vi "Wave2D_Cal U_Apply Corner.vi"(6 "time step":i32, 8 "y length":i32, 9 "x length":i32, 10 "Corner":T1, 11 "U In":dbl[][](array[numeric])) -> (3 "U Out":dbl[][](array[numeric]))   [LabVIEW 2020, in "NI_PDE.lvlib"]
uses:
  <vilib>/gmath/NI_PDE.lvlib
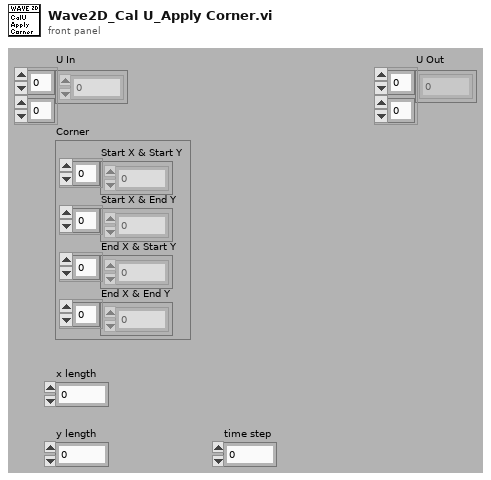
[diagram p1: front panel]
types:
  T1 = cluster{"Start X & Start Y":dbl[], "Start X & End Y":dbl[], "End X & Start Y":dbl[], "End X & End Y":dbl[]}
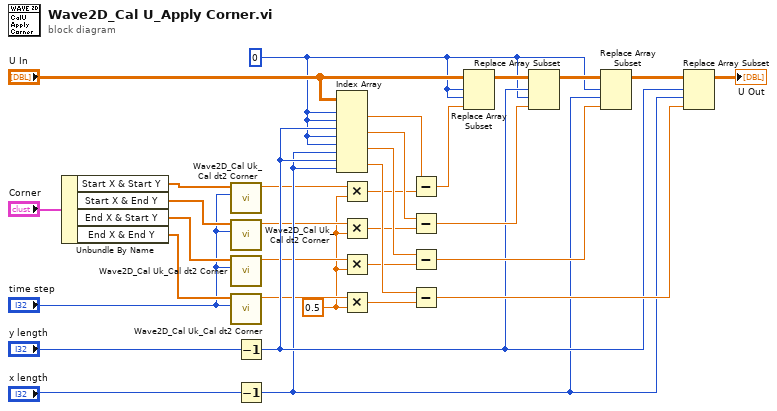
[diagram p0: block diagram]
diagram:
  w1 = 0.5 ("y")
  w11 = 0 ("index (row)")
  n1 = Unbundle By Name("Corner") -> ("Start X & Start Y"=w32:dbl[], "Start X & End Y"=w31:dbl[], "End X & Start Y"=w30:dbl[], "End X & End Y"=w29:dbl[])
  n2 = call <vilib>:"Wave2D_Cal Uk_Cal dt2 Corner.vi"("time step"="time step", "Corener"=w32) -> ("dt2 corner"=w9:dbl)  [unwired: 9 out]
  n3 = call <vilib>:"Wave2D_Cal Uk_Cal dt2 Corner.vi"("time step"="time step", "Corener"=w31) -> ("dt2 corner"=w7:dbl)  [unwired: 9 out]
  n4 = call <vilib>:"Wave2D_Cal Uk_Cal dt2 Corner.vi"("time step"="time step", "Corener"=w30) -> ("dt2 corner"=w5:dbl)  [unwired: 9 out]
  n5 = call <vilib>:"Wave2D_Cal Uk_Cal dt2 Corner.vi"("time step"="time step", "Corener"=w29) -> ("dt2 corner"=w3:dbl)  [unwired: 9 out]
  n6 = Decrement(x="y length") -> (x-1=w12:i32)
  n7 = Decrement(x="x length") -> (x-1=w10:i32)
  n8 = Index Array(array="U In", index (row) #1=w11, index (col) #1=w11, index (row) #2=w12, index (col) #2=w11, index (row) #3=w11, index (col) #3=w10, index (row) #4=w12, index (col) #4=w10) -> (element #1=w20:dbl, element #2=w18:dbl, element #3=w15:dbl, element #4=w14:dbl)
  n9 = Multiply(x=w9, y=w1) -> (x*y=w8:dbl)
  n10 = Multiply(x=w7, y=w1) -> (x*y=w6:dbl)
  n11 = Multiply(x=w5, y=w1) -> (x*y=w4:dbl)
  n12 = Multiply(x=w3, y=w1) -> (x*y=w2:dbl)
  n13 = Subtract(x=w20, y=w8) -> (x-y=w19:dbl)
  n14 = Subtract(x=w18, y=w6) -> (x-y=w17:dbl)
  n15 = Subtract(x=w15, y=w4) -> (x-y=w16:dbl)
  n16 = Subtract(x=w14, y=w2) -> (x-y=w13:dbl)
  n17 = Replace Array Subset(array="U In", new element=w19, index (row)=w11, index (col)=w11) -> (w27:dbl[][])
  n18 = Replace Array Subset(array=w27, new element=w17, index (row)=w12, index (col)=w11) -> (w24:dbl[][])
  n19 = Replace Array Subset(array=w24, new element=w16, index (row)=w11, index (col)=w10) -> (w23:dbl[][])
  n20 = Replace Array Subset(array=w23, new element=w13, index (row)=w12, index (col)=w10) -> (→"U Out":dbl[][])
